vi "StageMoveToEnd.vi"(6 "Velocity mm/s":sgl, 8 "error in (no error)":errorcluster, 9 "Target position mm":dbl=87.5 format="%_6g", 11 "Microscope in":refnum<class "Microscope.lvclass">) -> (0 "error out":errorcluster, 3 "Microscope out":refnum<class "Microscope.lvclass">)   [LabVIEW 2012, in "Microscope.lvclass"]
uses:
  classes/Microscope.lvclass
  classes/Microscope.lvclass/Microscope.ctl
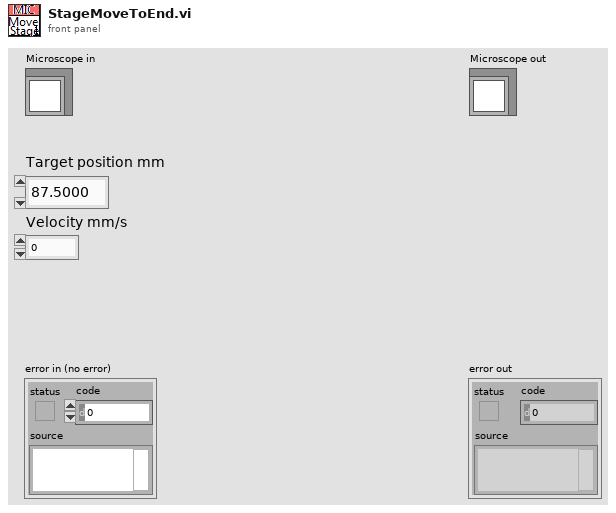
[diagram p1: front panel]
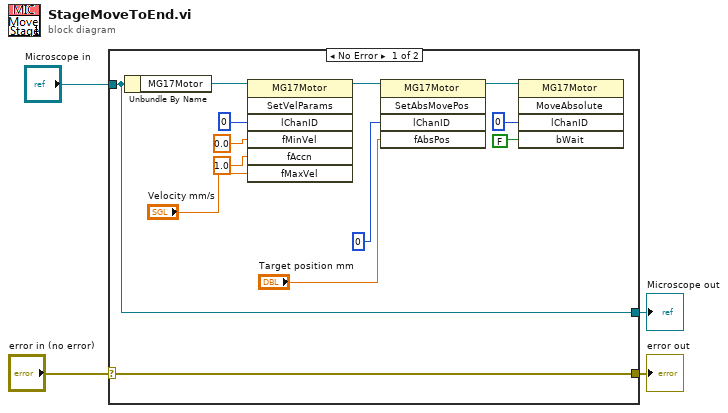
[diagram p0: block diagram]
diagram:
  n1 = case shown="No Error" "error in (no error)" {
    selector: "error in (no error)" -> [w17 w19]
    tunnel: [w17 w19] -> w3
    tunnel: [w7 w18] -> w1
    tunnel: "Microscope in" -> [w7 w18]
    frame No Error {
      n2 = Unbundle By Name(w7) -> ("MG17Motor"=w6:refnum<k7>)
      n3 = invoke class="MG17Motor" method="SetVelParams"(reference=w6, "lChanID"=0, "fMinVel"=sgl 0.0, "fAccn"=sgl 1.0, "fMaxVel"="Velocity mm/s") -> (reference out=w13:refnum<k7>)  [unwired: 2 in, 6 out]
      n4 = invoke class="MG17Motor" method="SetAbsMovePos"(reference=w13, "lChanID"=0, "fAbsPos"="Target position mm") -> (reference out=w14:refnum<k7>)  [unwired: 2 in, 4 out]
      n5 = invoke class="MG17Motor" method="MoveAbsolute"(reference=w14, "lChanID"=0, "bWait"=FALSE) -> ()  [unwired: 2 in, 5 out]
    }
    frame Error {
    }
  }
  "error out" <- w3
  "Microscope out" <- w1
